vi "laser1.0.vi"() -> ()   [LabVIEW 2019]
panel:
  out "Array":dbl[][](array[numeric])
  in  "Array 2":dbl[][](array[numeric])
  in  "Module_Path":path
  in  "Python_Version":string
  in  "Function_Name":string
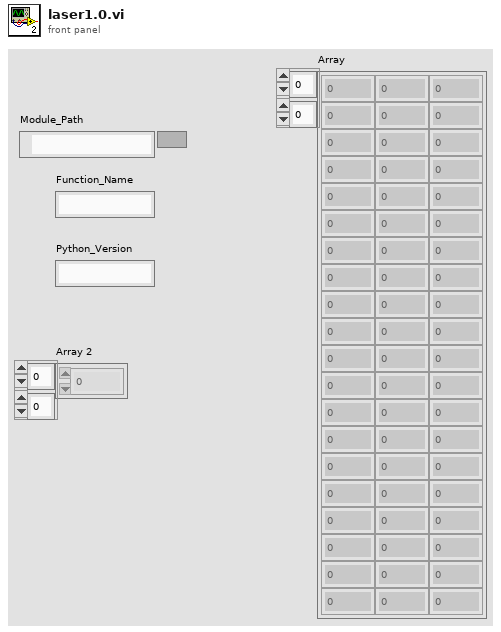
[diagram p1: front panel]
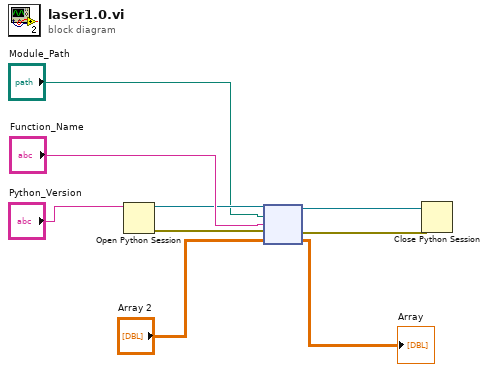
[diagram p0: block diagram]
diagram:
  n1 = Open Python Session(python version="Python_Version") -> (session out=w8:refnum<k35>, error out=w5:errorcluster)  [unwired: 2 in]
  n2 = node(w8, "Module_Path", "Function_Name", w5, "Array 2") -> (w7:refnum<k35>, w4:errorcluster, →"Array":dbl[][])  [unwired: 2 out]
  n3 = Close Python Session(session in=w7, error in=w4) -> ()  [unwired: 1 out]
